vi "[Teste]CaseSelect2.0.vi"() -> ()   [LabVIEW 2014]
panel:
  out "String":string
  in  "Voltagem":dbl
  in  "Condutividade":dbl
  out "Adsorção":bool
  in  "Liga/Desliga":bool
  out "Dessorção":bool
  out "Single-Pass":bool
  out "Batch":bool
  in  "BATCH / SINGLE PASS":bool
  in  "?":enum32{"POTENCIOSTÁTICO", "GALVANOSTÁTICO"}(tab)
  in  "Seletor de parâmetro P":enum32{"Tempo", "Condutividade"}(tab)
  in  "TEMPO DE ADSOR敲O P":dbl
  in  "TEMPO DE DESSOR敲O P":dbl
  in  "CONDUTIVIDADE \nMÍNIMA NA ADSORÇÃO P":dbl
  in  "CONDUTIVIDADE \nMÁXIMA NA DESSORÇÃO P":dbl
  in  "Selecionar parâmetro G":enum32{"Tempo", "Condutividade", "Potencial"}(tab)
  in  "TEMPO DE ADSOR敲O G":dbl
  in  "TEMPO DE DESSOR敲O G":dbl
  in  "CONDUTIVIDADE \nMÍNIMA NA ADSORÇÃO G":dbl
  in  "CONDUTIVIDADE \nMÁXIMA NA DESSORÇÃO G":dbl
  in  "POTENCIAL DE CORTE\nNA ADSOR敲O":dbl
  in  "POTENCIAL DE CORTE\nNA DESSOR敲O":dbl
  # "s"
  # "s"
  # "us/cm"
  # "us/cm"
  # "s"
  # "s"
  # "us/cm"
  # "us/cm"
  # "VV"
  # "V"
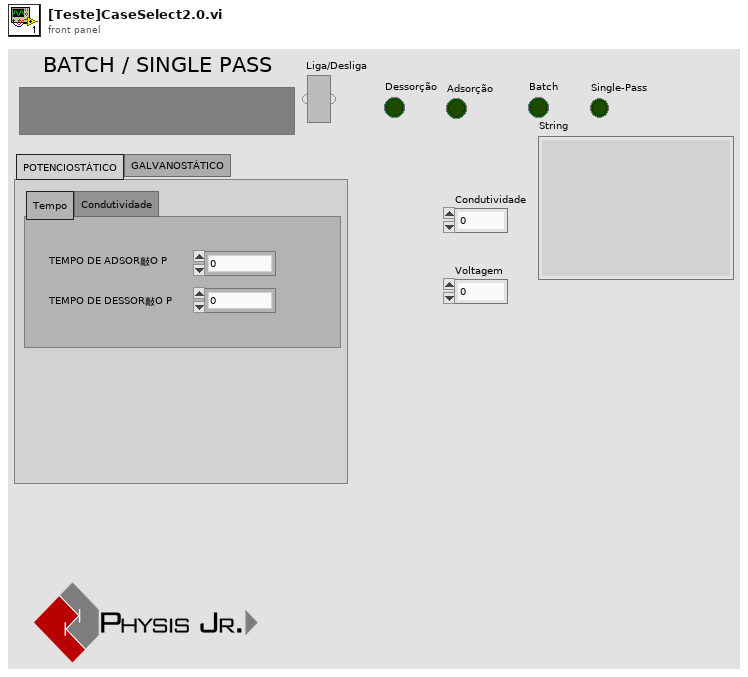
[diagram p1: front panel]
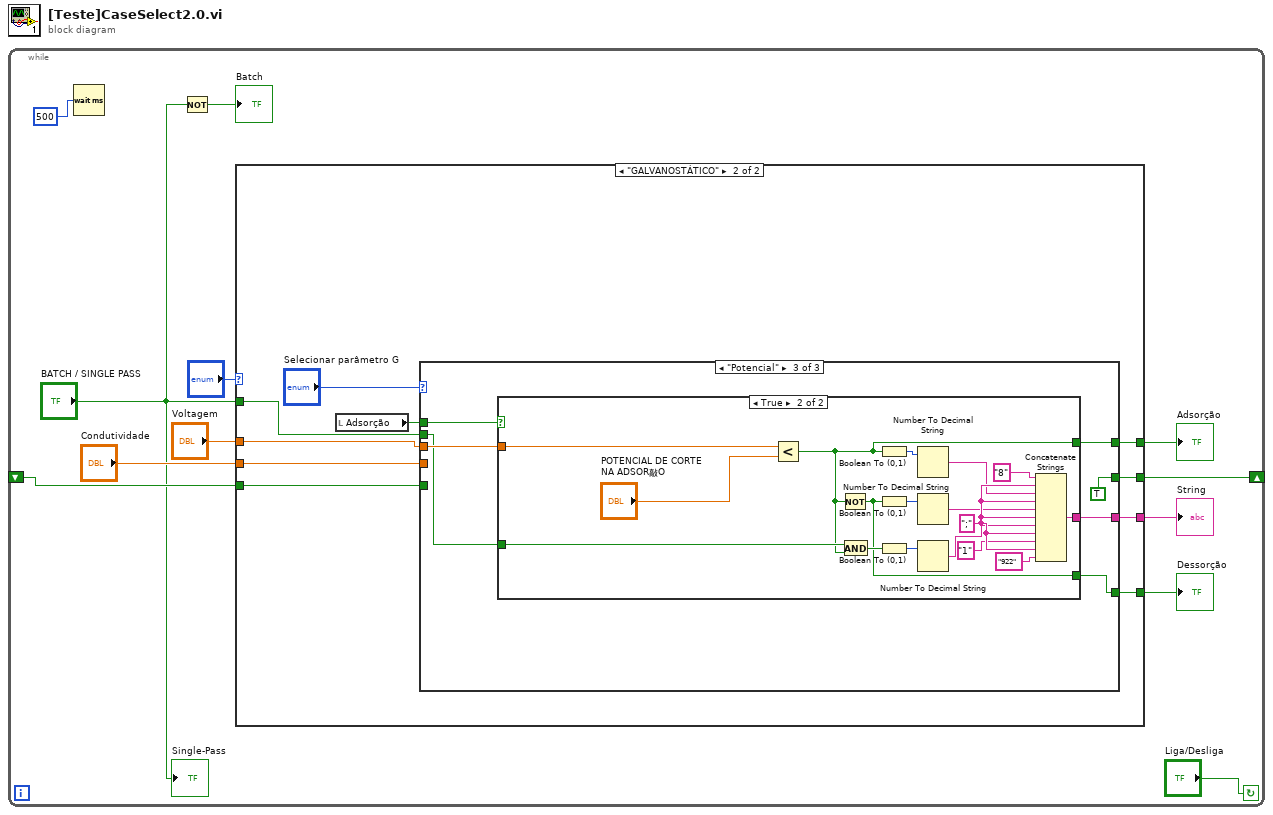
[diagram p0: block diagram]
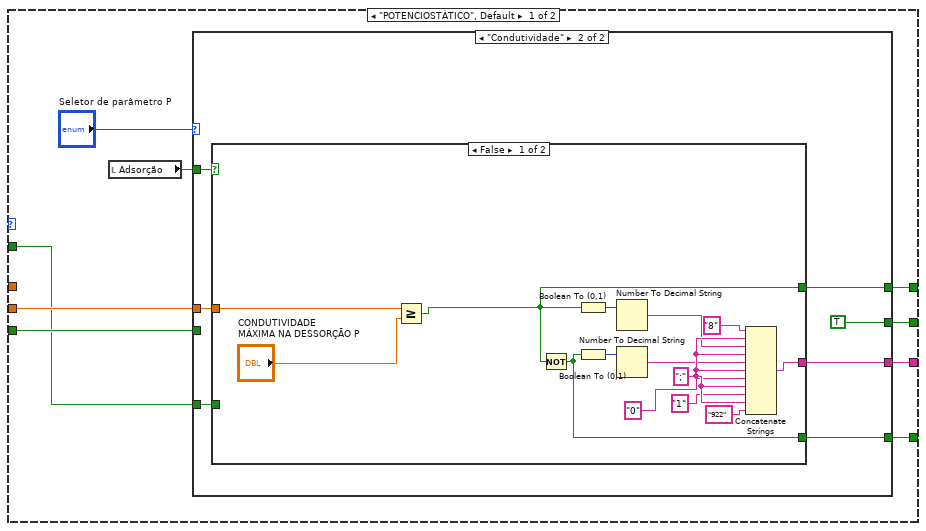
[diagram p2: hidden frame]
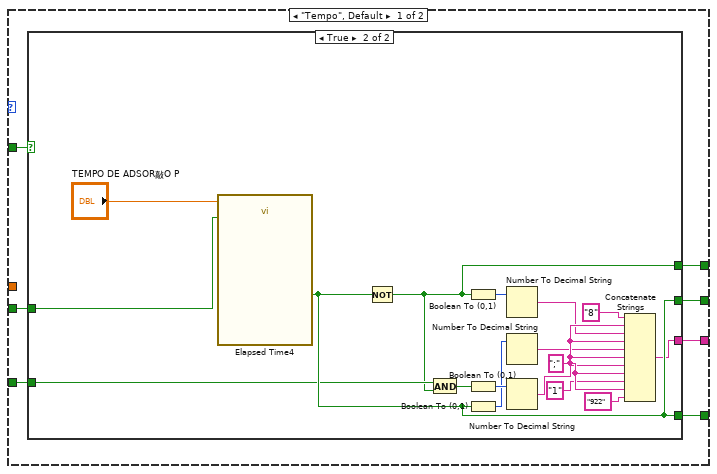
[diagram p3: hidden frame]
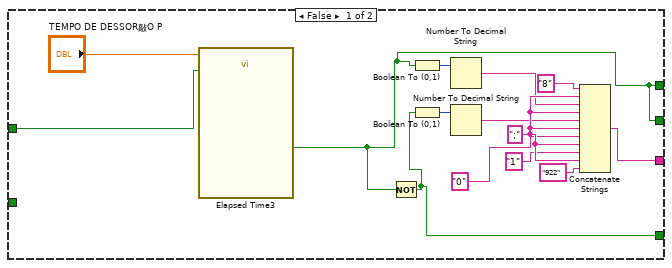
[diagram p4: hidden frame]
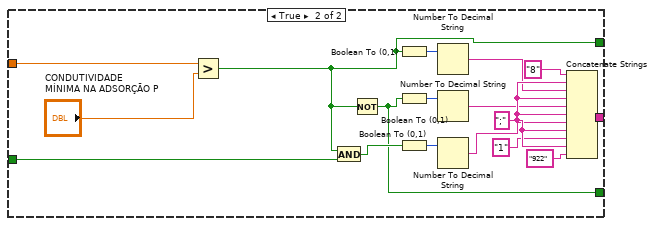
[diagram p5: hidden frame]
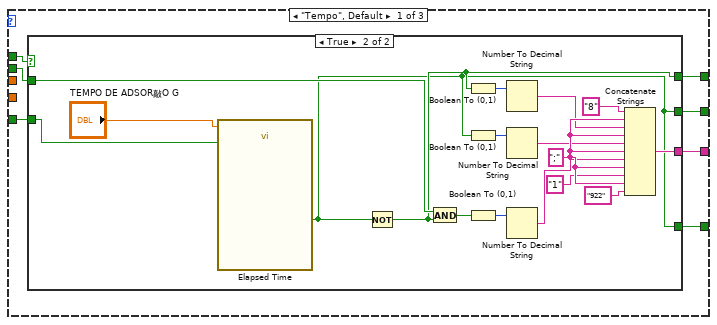
[diagram p6: hidden frame]
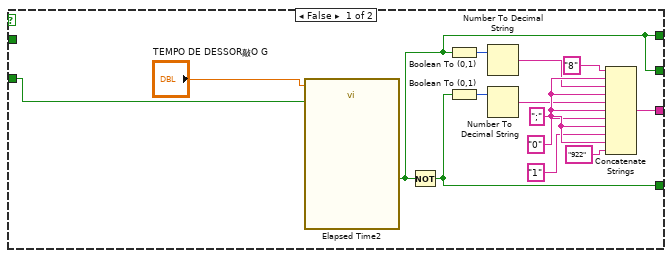
[diagram p7: hidden frame]
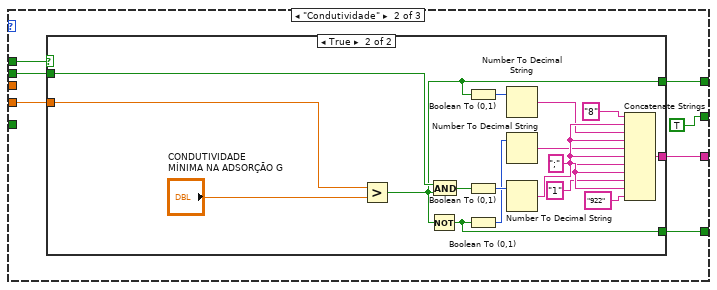
[diagram p8: hidden frame]
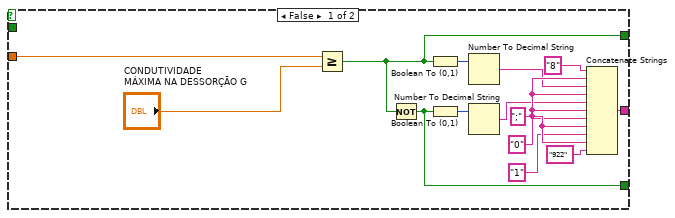
[diagram p9: hidden frame]
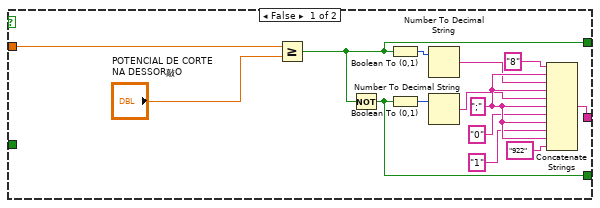
[diagram p10: hidden frame]
diagram:
  n1 = while {
    shift-right: [w7] -> _
    shift-left: _ -> [w8]
    stop <- "Liga/Desliga" continue-if-true
    n2 = Wait (ms)(milliseconds to wait=500) -> ()  [unwired: 1 out]
    n3 = Not(x="BATCH / SINGLE PASS") -> (.not. x?=→"Batch":bool)
    n4 = case shown="\"GALVANOSTÁTICO\"" "?" {
      tunnel: "Voltagem" -> [_ w105]
      tunnel: "Condutividade" -> [w19 w104]
      tunnel: w8 -> [w18 w103]
      tunnel: [w17 w102] -> w7
      tunnel: [w16 w101] -> w5
      tunnel: [w15 w100] -> w4
      tunnel: [w13 w99] -> w3
      tunnel: "BATCH / SINGLE PASS" -> [w14 w98]
      frame "POTENCIOSTÁTICO", Default {
        n5 = local read "Adsorção"() -> (w20:bool)
        n6 = case shown="\"Condutividade\"" "Seletor de parâmetro P" {
          tunnel: w20 -> [w28 w66]
          tunnel: w19 -> [_ w65]
          tunnel: w18 -> [w27 _]
          tunnel: [w26 TRUE] -> w17
          tunnel: [w25 w63] -> w16
          tunnel: [w24 w62] -> w15
          tunnel: w14 -> [w23 w61]
          tunnel: [w22 w64] -> w13
          frame "Tempo", Default {
            n7 = case shown="True" w28 {
              tunnel: w27 -> [w41 w58]
              tunnel: [w29 w47] -> w26
              tunnel: [w29 w45] -> w25
              tunnel: [w30 w47] -> w24
              tunnel: w23 -> [_ w46]
              tunnel: [w31 w43] -> w22
              frame False {
                w38 = ";"
                n8 = call "Elapsed Time3"("Time Target (s)"="TEMPO DE DESSOR敲O P", "Reset"=w41) -> ("Time has Elapsed"=w29:bool)  [unwired: 10 in, 7 out]
                n9 = Not(x=w29) -> (.not. x?=w30:bool)
                n10 = Boolean To (0,1)(Boolean=w29) -> (0, 1=w37:i16)
                n11 = Boolean To (0,1)(Boolean=w30) -> (0, 1=w36:i16)
                n12 = Number To Decimal String(number=w37) -> (decimal integer string=w34:string)  [unwired: 1 in]
                n13 = Number To Decimal String(number=w36) -> (decimal integer string=w35:string)  [unwired: 1 in]
                n14 = Concatenate Strings("8", w38, w34, w38, w35, w38, "0", w38, "1", w38, "922") -> (w31:string)
              }
              frame True {
                w54 = ";"
                n15 = call "Elapsed Time4"("Time Target (s)"="TEMPO DE ADSOR敲O P", "Reset"=w58) -> ("Time has Elapsed"=w47:bool)  [unwired: 10 in, 7 out]
                n16 = Not(x=w47) -> (.not. x?=w45:bool)
                n17 = And(x=w46, y=w45) -> (x .and. y?=w44:bool)
                n18 = Boolean To (0,1)(Boolean=w45) -> (0, 1=w53:i16)
                n19 = Boolean To (0,1)(Boolean=w44) -> (0, 1=w57:i16)
                n20 = Boolean To (0,1)(Boolean=w47) -> (0, 1=w52:i16)
                n21 = Number To Decimal String(number=w53) -> (decimal integer string=w50:string)  [unwired: 1 in]
                n22 = Number To Decimal String(number=w52) -> (decimal integer string=w51:string)  [unwired: 1 in]
                n23 = Number To Decimal String(number=w57) -> (decimal integer string=w49:string)  [unwired: 1 in]
                n24 = Concatenate Strings("8", w54, w50, w54, w51, w54, w49, w54, "1", w54, "922") -> (w43:string)
              }
            }
          }
          frame "Condutividade" {
            n25 = case shown="False" w66 {
              tunnel: w65 -> [w80 w97]
              tunnel: [w70 w81] -> w64
              tunnel: [w69 w83] -> w63
              tunnel: [w68 w82] -> w62
              tunnel: w61 -> [_ w85]
              frame False {
                w76 = ";"
                n26 = Greater Or Equal?(x=w80, y="CONDUTIVIDADE \nMÁXIMA NA DESSORÇÃO P") -> (x >= y?=w69:bool)
                n27 = Not(x=w69) -> (.not. x?=w68:bool)
                n28 = Boolean To (0,1)(Boolean=w69) -> (0, 1=w75:i16)
                n29 = Boolean To (0,1)(Boolean=w68) -> (0, 1=w74:i16)
                n30 = Number To Decimal String(number=w75) -> (decimal integer string=w72:string)  [unwired: 1 in]
                n31 = Number To Decimal String(number=w74) -> (decimal integer string=w73:string)  [unwired: 1 in]
                n32 = Concatenate Strings("8", w76, w72, w76, w73, w76, "0", w76, "1", w76, "922") -> (w70:string)
              }
              frame True {
                w92 = ";"
                n33 = Greater?(x=w97, y="CONDUTIVIDADE \nMÍNIMA NA ADSORÇÃO P") -> (0:w83:bool)
                n34 = And(x=w83, y=w85) -> (x .and. y?=w84:bool)
                n35 = Not(x=w83) -> (.not. x?=w82:bool)
                n36 = Boolean To (0,1)(Boolean=w83) -> (0, 1=w91:i16)
                n37 = Boolean To (0,1)(Boolean=w82) -> (0, 1=w90:i16)
                n38 = Boolean To (0,1)(Boolean=w84) -> (0, 1=w95:i16)
                n39 = Number To Decimal String(number=w91) -> (decimal integer string=w88:string)  [unwired: 1 in]
                n40 = Number To Decimal String(number=w90) -> (decimal integer string=w89:string)  [unwired: 1 in]
                n41 = Number To Decimal String(number=w95) -> (decimal integer string=w87:string)  [unwired: 1 in]
                n42 = Concatenate Strings("8", w92, w88, w92, w89, w92, w87, w92, "1", w92, "922") -> (w81:string)
              }
            }
          }
        }
      }
      frame "GALVANOSTÁTICO" {
        n43 = local read "Adsorção"() -> (w106:bool)
        n44 = case shown="\"Potencial\"" "Selecionar parâmetro G" {
          tunnel: w106 -> [w114 w152 w190]
          tunnel: w105 -> [_ _ w189]
          tunnel: w104 -> [_ w151 _]
          tunnel: w103 -> [w113 _ _]
          tunnel: [w112 TRUE TRUE] -> w102
          tunnel: [w111 w148 w186] -> w101
          tunnel: [w110 w147 w185] -> w100
          tunnel: [w109 w150 w187] -> w99
          tunnel: w98 -> [w108 w149 w188]
          frame "Tempo", Default {
            n45 = case shown="True" w114 {
              tunnel: w113 -> [w127 w144]
              tunnel: [w118 w129] -> w112
              tunnel: [w118 w132] -> w111
              tunnel: [w117 w129] -> w110
              tunnel: [w115 w130] -> w109
              tunnel: w108 -> [_ w133]
              frame False {
                w124 = ";"
                n46 = call "Elapsed Time2"("Time Target (s)"="TEMPO DE DESSOR敲O G", "Reset"=w127) -> ("Time has Elapsed"=w118:bool)  [unwired: 10 in, 7 out]
                n47 = Not(x=w118) -> (.not. x?=w117:bool)
                n48 = Boolean To (0,1)(Boolean=w118) -> (0, 1=w123:i16)
                n49 = Boolean To (0,1)(Boolean=w117) -> (0, 1=w122:i16)
                n50 = Number To Decimal String(number=w123) -> (decimal integer string=w120:string)  [unwired: 1 in]
                n51 = Number To Decimal String(number=w122) -> (decimal integer string=w121:string)  [unwired: 1 in]
                n52 = Concatenate Strings("8", w124, w120, w124, w121, w124, "0", w124, "1", w124, "922") -> (w115:string)
              }
              frame True {
                w140 = ";"
                n53 = call "Elapsed Time"("Time Target (s)"="TEMPO DE ADSOR敲O G", "Reset"=w144) -> ("Time has Elapsed"=w129:bool)  [unwired: 10 in, 7 out]
                n54 = Not(x=w129) -> (.not. x?=w132:bool)
                n55 = And(x=w133, y=w132) -> (x .and. y?=w131:bool)
                n56 = Boolean To (0,1)(Boolean=w132) -> (0, 1=w139:i16)
                n57 = Boolean To (0,1)(Boolean=w129) -> (0, 1=w138:i16)
                n58 = Boolean To (0,1)(Boolean=w131) -> (0, 1=w143:i16)
                n59 = Number To Decimal String(number=w139) -> (decimal integer string=w136:string)  [unwired: 1 in]
                n60 = Number To Decimal String(number=w138) -> (decimal integer string=w137:string)  [unwired: 1 in]
                n61 = Number To Decimal String(number=w143) -> (decimal integer string=w135:string)  [unwired: 1 in]
                n62 = Concatenate Strings("8", w140, w136, w140, w137, w140, w135, w140, "1", w140, "922") -> (w130:string)
              }
            }
          }
          frame "Condutividade" {
            n63 = case shown="True" w152 {
              tunnel: w151 -> [w166 w183]
              tunnel: [w155 w171] -> w150
              tunnel: w149 -> [_ w169]
              tunnel: [w154 w168] -> w148
              tunnel: [w153 w167] -> w147
              frame False {
                w162 = ";"
                n64 = Greater Or Equal?(x=w166, y="CONDUTIVIDADE \nMÁXIMA NA DESSORÇÃO G") -> (x >= y?=w154:bool)
                n65 = Not(x=w154) -> (.not. x?=w153:bool)
                n66 = Boolean To (0,1)(Boolean=w154) -> (0, 1=w161:i16)
                n67 = Boolean To (0,1)(Boolean=w153) -> (0, 1=w160:i16)
                n68 = Number To Decimal String(number=w161) -> (decimal integer string=w158:string)  [unwired: 1 in]
                n69 = Number To Decimal String(number=w160) -> (decimal integer string=w159:string)  [unwired: 1 in]
                n70 = Concatenate Strings("8", w162, w158, w162, w159, w162, "0", w162, "1", w162, "922") -> (w155:string)
              }
              frame True {
                w178 = ";"
                n71 = Greater?(x=w183, y="CONDUTIVIDADE \nMÍNIMA NA ADSORÇÃO G") -> (0:w168:bool)
                n72 = Not(x=w168) -> (.not. x?=w167:bool)
                n73 = And(x=w169, y=w168) -> (x .and. y?=w170:bool)
                n74 = Boolean To (0,1)(Boolean=w168) -> (0, 1=w177:i16)
                n75 = Boolean To (0,1)(Boolean=w170) -> (0, 1=w181:i16)
                n76 = Boolean To (0,1)(Boolean=w167) -> (0, 1=w176:i16)
                n77 = Number To Decimal String(number=w177) -> (decimal integer string=w174:string)  [unwired: 1 in]
                n78 = Number To Decimal String(number=w176) -> (decimal integer string=w175:string)  [unwired: 1 in]
                n79 = Number To Decimal String(number=w181) -> (decimal integer string=w173:string)  [unwired: 1 in]
                n80 = Concatenate Strings("8", w178, w174, w178, w175, w178, w173, w178, "1", w178, "922") -> (w171:string)
              }
            }
          }
          frame "Potencial" {
            n81 = case shown="True" w190 {
              tunnel: w189 -> [w204 w221]
              tunnel: w188 -> [_ w208]
              tunnel: [w193 w207] -> w187
              tunnel: [w192 w206] -> w186
              tunnel: [w191 w205] -> w185
              frame False {
                w200 = ";"
                n82 = Greater Or Equal?(x=w204, y="POTENCIAL DE CORTE\nNA DESSOR敲O") -> (x >= y?=w192:bool)
                n83 = Not(x=w192) -> (.not. x?=w191:bool)
                n84 = Boolean To (0,1)(Boolean=w192) -> (0, 1=w199:i16)
                n85 = Boolean To (0,1)(Boolean=w191) -> (0, 1=w198:i16)
                n86 = Number To Decimal String(number=w199) -> (decimal integer string=w196:string)  [unwired: 1 in]
                n87 = Number To Decimal String(number=w198) -> (decimal integer string=w197:string)  [unwired: 1 in]
                n88 = Concatenate Strings("8", w200, w196, w200, w197, w200, "0", w200, "1", w200, "922") -> (w193:string)
              }
              frame True {
                w216 = ";"
                n89 = Less?(x=w221, y="POTENCIAL DE CORTE\nNA ADSOR敲O") -> (x < y?=w206:bool)
                n90 = Not(x=w206) -> (.not. x?=w205:bool)
                n91 = And(x=w208, y=w206) -> (x .and. y?=w209:bool)
                n92 = Boolean To (0,1)(Boolean=w206) -> (0, 1=w215:i16)
                n93 = Boolean To (0,1)(Boolean=w205) -> (0, 1=w214:i16)
                n94 = Boolean To (0,1)(Boolean=w209) -> (0, 1=w219:i16)
                n95 = Number To Decimal String(number=w215) -> (decimal integer string=w212:string)  [unwired: 1 in]
                n96 = Number To Decimal String(number=w214) -> (decimal integer string=w213:string)  [unwired: 1 in]
                n97 = Number To Decimal String(number=w219) -> (decimal integer string=w211:string)  [unwired: 1 in]
                n98 = Concatenate Strings("8", w216, w212, w216, w213, w216, w211, w216, "1", w216, "922") -> (w207:string)
              }
            }
          }
        }
      }
    }
    "Dessorção" <- w4
    "Adsorção" <- w5
    "String" <- w3
    "Single-Pass" <- "BATCH / SINGLE PASS"
  }
